vi "Close.vi"(8 "error in (no error)":errorcluster, 10 "Reason":T1, 11 "Panel in":refnum<class "Panel.lvclass">) -> (0 "error out":errorcluster, 3 "Panel out":refnum<class "Panel.lvclass">)   [LabVIEW 2020, in "OOPanel.lvlib" / "Panel.lvclass"]
uses:
  Panel.lvclass
  Close Reason.ctl
  Panel.lvclass/Panel.ctl
  OOPanel.lvlib
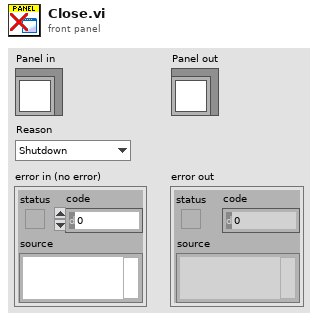
[diagram p1: front panel]
types:
  T1 = typedef "OOPanel.lvlib/Close Reason.ctl" = enum16{"Shutdown", "Close"}
  T2 = typedef "OOPanel.lvlib/Panel.lvclass/Ref Data.ctl" = cluster{"Panel Ref":refnum<vi>, "SubPanel":refnum<vi>, "Close":bool, "Running":bool, "State":T3}
  T3 = typedef "OOPanel.lvlib/Visibility State.ctl" = enum16{"Idle", "Closed", "Hidden", "Visible", "Subpanel", "Hidden Subpanel"}
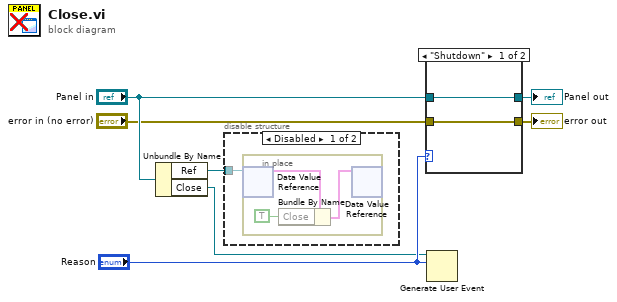
[diagram p0: block diagram]
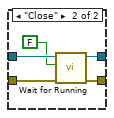
[diagram p3: hidden frame]
diagram:
  n1 = Unbundle By Name("Panel in") -> ("Ref"=w7:refnum<data-value>, "Close"=w1:refnum<user-event>)
  n2 = disable-structure shown="Disabled" {
    disable-tunnel: w7 -> [w8 _]
    frame Disabled {
      n3 = in-place {
        n4 = in-place-dvr #1(w8) -> (w11:T2)  [unwired: 1 out]
        n5 = Bundle By Name(cluster=w11, "Close"=TRUE) -> (w9:T2)
        n6 = in-place-dvr #1(w9) -> ()  [unwired: 2 out]
      }
    }
    frame Enabled {
    }
  }
  n7 = case shown="\"Shutdown\"" "Reason" {
    tunnel: "Panel in" -> [w13 w18]
    tunnel: "error in (no error)" -> [w12 w17]
    tunnel: [w12 w15] -> w4
    tunnel: [w13 w14] -> w3
    frame "Shutdown" {
    }
    frame "Close" {
      n8 = call "Wait for Running.vi"("error in (no error)"=w17, "Running"=FALSE, "Panel in"=w18) -> ("error out"=w15:errorcluster, "Panel out"=w14:refnum<class "Panel.lvclass">)  [unwired: 7 in]
    }
  }
  "error out" <- w4
  "Panel out" <- w3
  n9 = Generate User Event(user event=w1, event data cluster="Reason") -> ()  [unwired: 2 in, 2 out]
